vi "Create Shared Variables.vi"(8 "error in":errorcluster, 9 "Data Type":variant, 10 "Variable Names":string[](array[string])) -> (0 "error out":errorcluster)   [LabVIEW 2017, in "Shared Variables Library.lvlib"]
doc: "Adds shared variables to a container (the library file defined by the constant) and then deploys those variables, so that they are available to other applications."
uses:
  Shared Variables Library.lvlib
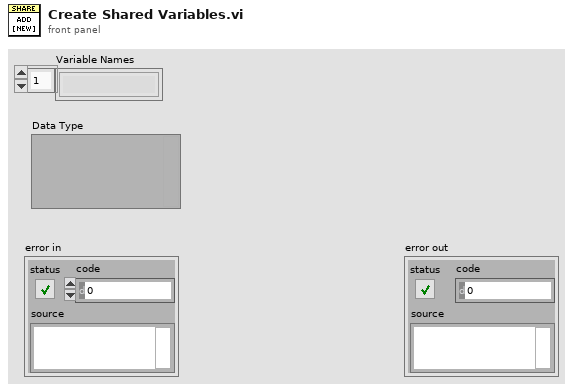
[diagram p1: front panel]
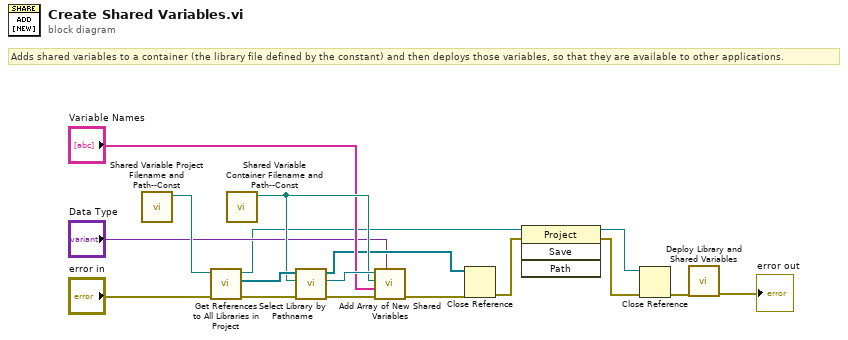
[diagram p0: block diagram]
diagram:
  # "Adds shared variables to a container (the library file defined by the constant) and then deploys those variables, so that they are available to other applications."
  n1 = call "Shared Variable Project Filename and Path--Const.vi"() -> ("appended path"=w17:path)  [unwired: 11 in]
  n2 = call "Get References to All Libraries in Project.vi"("error in"="error in", "Project Path"=w17) -> ("error out"=w14:errorcluster, "All Libraries"=w15:refnum<vi>[], "Project Reference"=w6:refnum<vi>)  [unwired: 7 in]
  n3 = call "Shared Variable Container Filename and Path--Const.vi"() -> ("Path to Shared Variable Containing Library"=w12:path)  [unwired: 11 in]
  n4 = call "Select Library by Pathname.vi"("error in"=w14, "Path to Library"=w12, "All Libraries In"=w15) -> ("error out"=w16:errorcluster, "Selected Library"=w13:refnum<vi>, "All Libraries Out"=w10:refnum<vi>[])  [unwired: 6 in]
  n5 = call "Add Array of New Shared Variables.vi"("Data Type (Variant)"="Data Type", "error in"=w16, "Variable Names"="Variable Names", "Library Path"=w12, "Selected Library In"=w13) -> ("error out"=w9:errorcluster)  [unwired: 5 in, 1 out]
  n6 = Close Reference(reference=w10, error in (no error)=w9) -> (error out=w5:errorcluster)
  n7 = invoke class="Project" method="Save"(reference=w6, error in=w5) -> (reference out=w4:refnum<vi>, error out=w3:errorcluster)  [unwired: 2 in, 2 out]
  n8 = Close Reference(reference=w4, error in (no error)=w3) -> (error out=w2:errorcluster)
  n9 = call "Deploy Library and Shared Variables.vi"("error in"=w2) -> ("error out"=→"error out":errorcluster)  [unwired: 10 in]
